vi "zad3.vi"() -> ()   [LabVIEW 2017]
panel:
  out "Numeric 2":dbl
  out "Numeric":dbl
  in  "Prąd [mA]":dbl min=0.0 max=1.1
  in  "TRYB":i16(knob) step=1 scale=1.0..3.0
  in  "DAC0":dbl(knob) scale=0.04..2.5
  out "Rs":dbl
  in  "Interval (ms)":u32=500
  in  "stop":bool
  out "AIN3":dbl format="%.6f"
  out "AIN2":dbl format="%.6f"
  out "Error Message":string
  out "error out":errorcluster
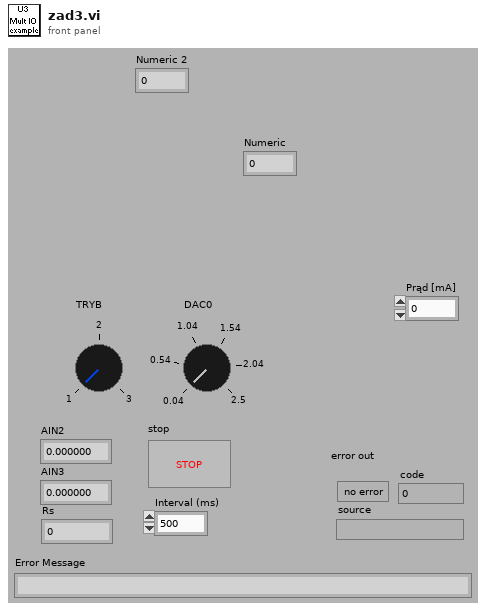
[diagram p1: front panel]
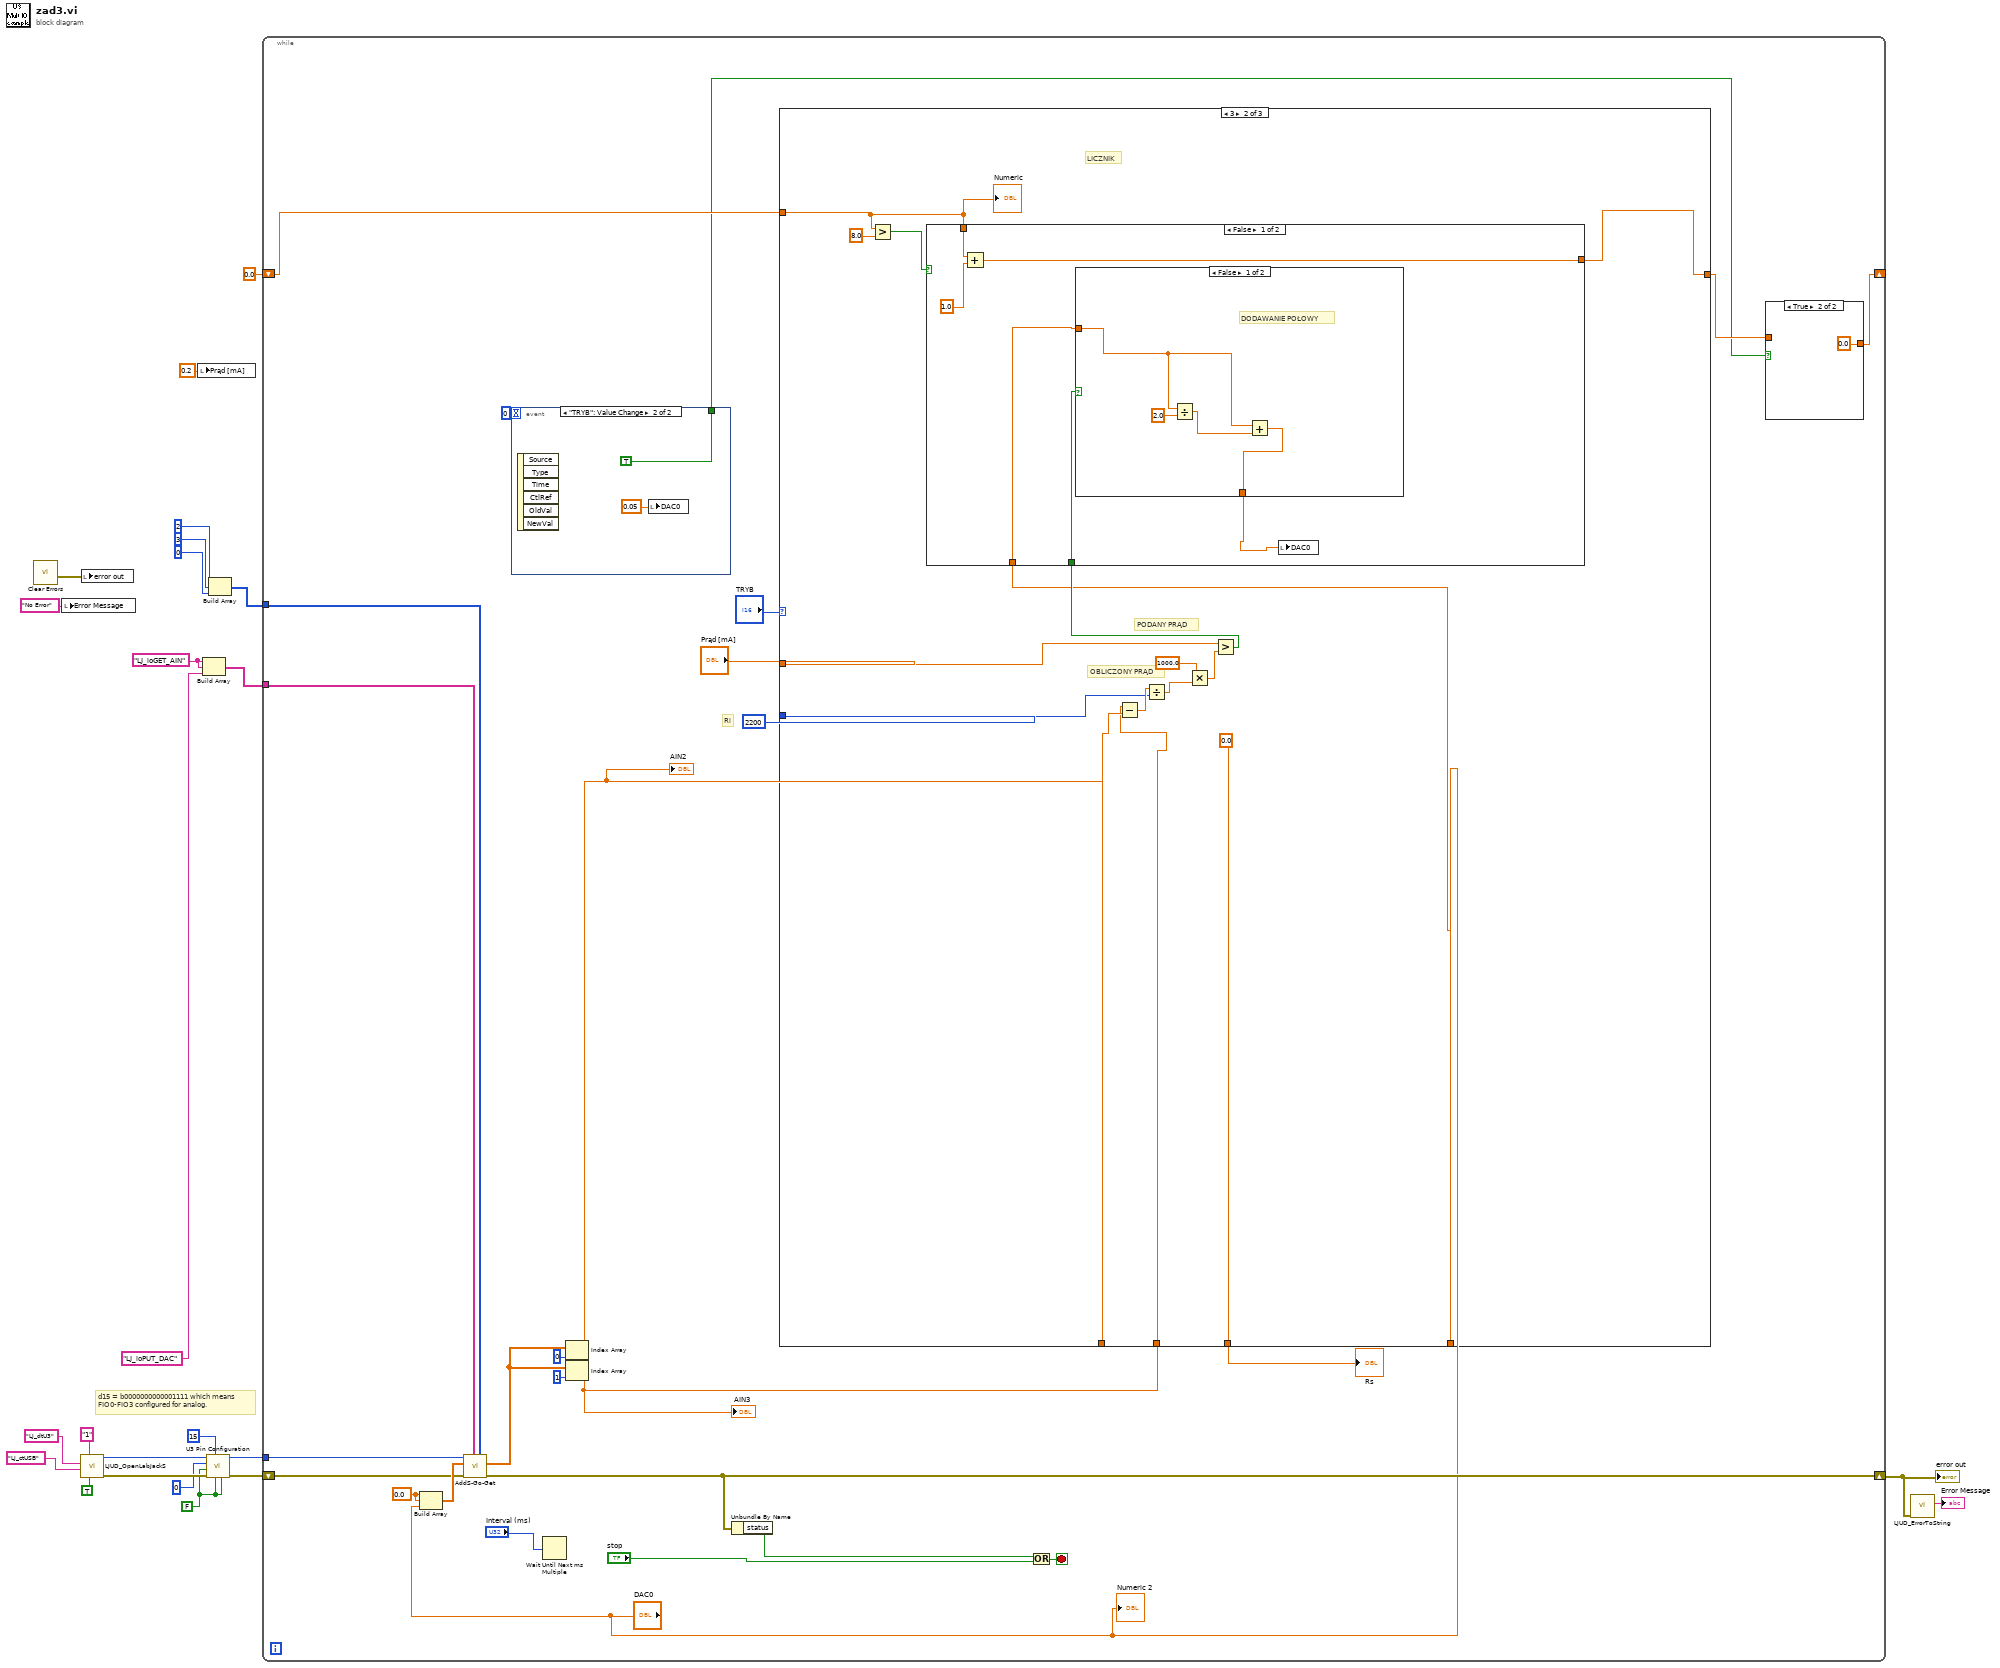
[diagram p0: block diagram]
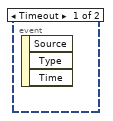
[diagram p3: hidden frame]
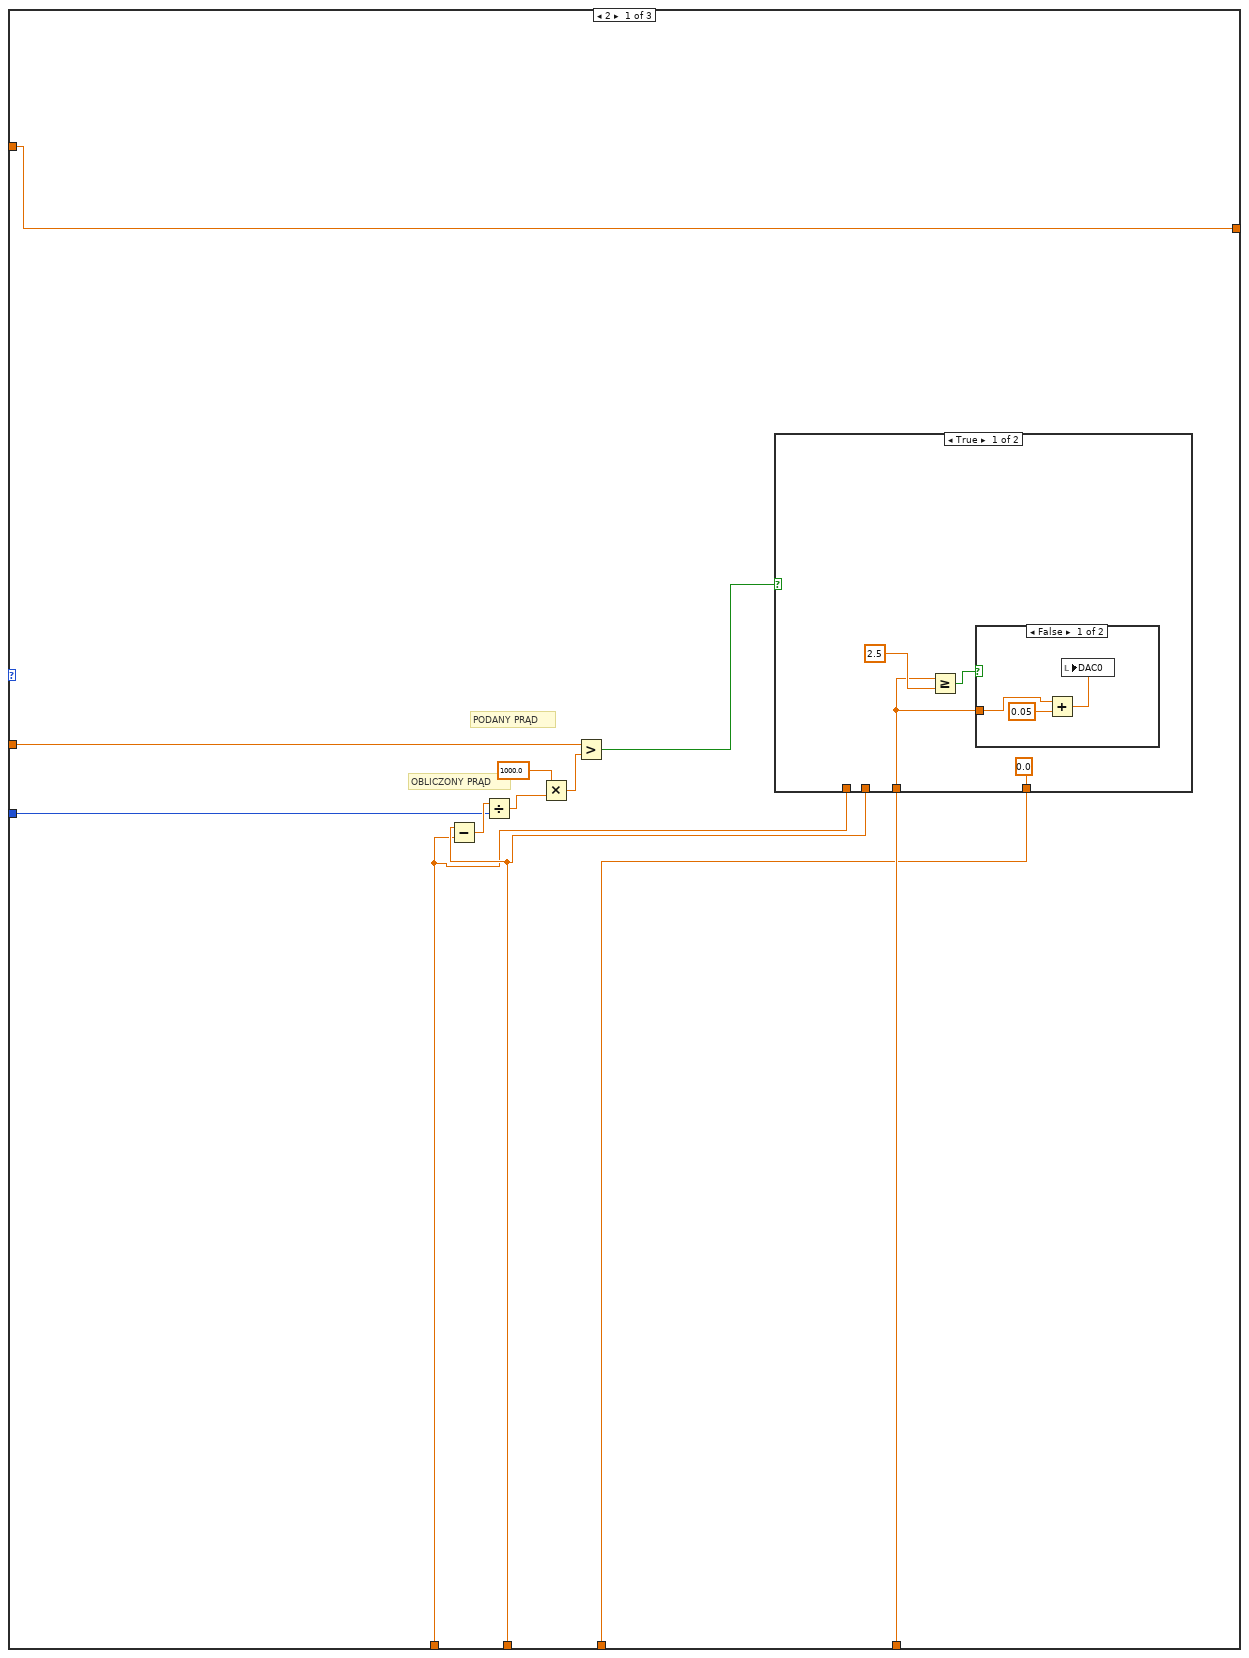
[diagram p4: hidden frame]
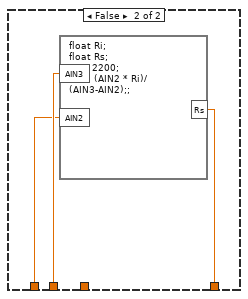
[diagram p6: hidden frame]
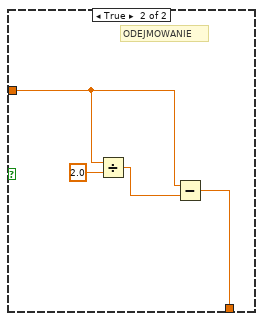
[diagram p7: hidden frame]
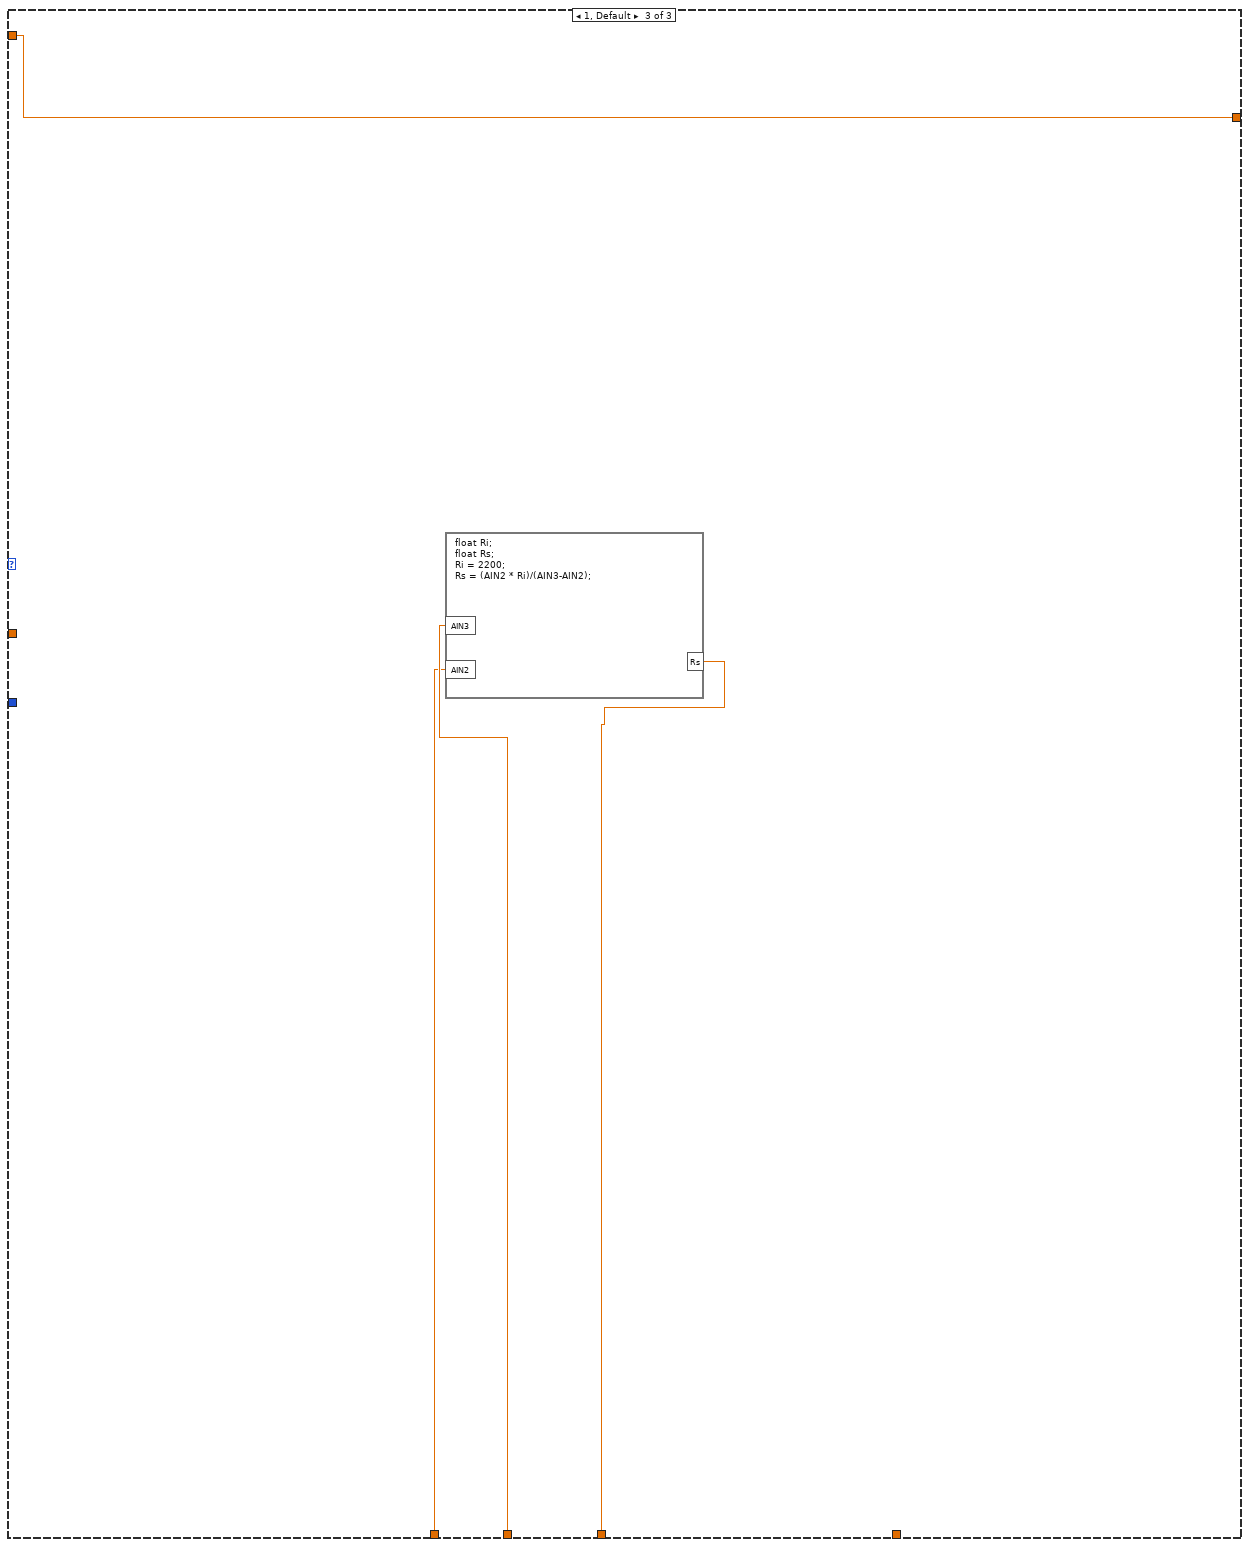
[diagram p9: hidden frame]
diagram:
  w7 = FALSE ("Enable DAC1")
  w3 = "LJ_ioGET_AIN" ("IOType")
  # "d15 = b0000000000001111 which means\nFIO0-FIO3 configured for analog."
  n1 = call <vilib>:"Clear Errors.vi"() -> ("error out"=w5:errorcluster)  [unwired: 6 in, 1 out]
  n2 = local write "Error Message"("No Error" ("Error Message")) -> ()
  n3 = call "LJUD_OpenLabJackS.vi"("FirstFound"=TRUE, "Address"="1", "ConnectionType"="LJ_ctUSB", "DeviceType"="LJ_dtU3") -> ("error out"=w12:errorcluster, "Handle"=w10:i32)  [unwired: 5 in, 1 out]
  n4 = local write "error out"(w5) -> ()
  n5 = local write "Prąd [mA]"(0.2 ("Prąd [A]")) -> ()
  n6 = Build Array(w3, w3, "LJ_ioPUT_DAC" ("IOType")) -> (w23:string[])
  n7 = call "U3 Pin Configuration.vi"("Enable Counter1"=w7, "Enable Counter0"=w7, "FIO/EIO Analog Enable"=15, "error in"=w12, "Enable DAC1"=w7, "Number of Timers Enabled"=u8 0, "Handle In"=w10) -> ("error out"=w13:errorcluster, "Handle Out"=w11:i32)  [unwired: 3 in]
  n8 = Build Array(2, 3, 0) -> (w22:i32[])
  n9 = while {
    shift-left: w13 -> [w39]
    shift-right: [w38] -> w14
    tunnel: w11 -> [w43]
    tunnel: w22 -> [w49]
    tunnel: w23 -> [w50]
    shift-right: [w27] -> _
    shift-left: 0.0 -> [w29]
    stop <- w42 stop-if-true
    w48 = 0.0 ("Input Element")
    # "Ri"
    n10 = Build Array(w48, w48, "DAC0") -> (w47:dbl[])
    n11 = call "AddS-Go-Get.vi"("Channels"=w49, "IOTypes"=w50, "error in"=w39, "Values Write"=w47, "Handle In"=w43) -> ("error out"=w38:errorcluster, "Values Read"=w44:dbl[])  [unwired: 4 in, 1 out]
    n12 = event shown="[1] \"TRYB\": Value Change" {
      selector: _ -> [_ _]
      dyn-events: _ -> [_ _]
      timeout: 0 -> [_ _]
      tunnel: [_ TRUE] -> w26
      event Timeout {
        n13 = event-data() -> ()  [unwired: 1 in, 3 out]
      }
      event "TRYB": Value Change {
        n14 = event-data() -> ()  [unwired: 1 in, 6 out]
        n15 = local write "DAC0"(0.05 ("DAC0")) -> ()
      }
    }
    n16 = Wait Until Next ms Multiple(millisecond multiple="Interval (ms)") -> ()  [unwired: 1 out]
    n17 = Index Array(array=w44, index=0 ("Index")) -> (element=w35:dbl)
    "AIN2" <- w35
    n18 = Index Array(array=w44, index=1 ("Index")) -> (element=w36:dbl)
    "AIN3" <- w36
    n19 = Unbundle By Name(w38) -> ("status"=w40:bool)
    n20 = case shown="3" "TRYB" {
      tunnel: w36 -> [w62 w85 w110]
      tunnel: w35 -> [w61 w86 w109]
      tunnel: [w60 0.0 w108] -> w34
      tunnel: 2200 -> [w65 w87 _]
      tunnel: "DAC0" -> [w63 w78 _]
      tunnel: "Prąd [mA]" -> [w56 w83 _]
      tunnel: [w55 w80 w107] -> w28
      tunnel: w29 -> [w55 w81 w107]
      frame 2 {
        # "PODANY PRĄD"
        # "OBLICZONY PRĄD"
        n21 = Subtract(x=w62, y=w61) -> (x-y=w66:dbl)
        n22 = Divide(x=w66, y=w65) -> (x/y=w59:dbl)
        n23 = Multiply(x=1000.0, y=w59) -> (x*y=w57:dbl)
        n24 = Greater?(x=w56, y=w57) -> (0:w64:bool)
        n25 = case shown="True" w64 {
          tunnel: w63 -> [w68 _]
          tunnel: w62 -> [_ w76]
          tunnel: w61 -> [_ w75]
          tunnel: [0.0 w74] -> w60
          frame True {
            n26 = Greater Or Equal?(x=w68, y=2.5) -> (x >= y?=w69:bool)
            n27 = case shown="False" w69 {
              tunnel: w68 -> [w71 _]
              frame False {
                n28 = Add(x=w71, y=0.05) -> (x+y=w73:dbl)
                n29 = local write "DAC0"(w73) -> ()
              }
              frame True {
              }
            }
          }
          frame False {
            n30 = formula code="float Ri;\nfloat Rs;\nRi = 2200;\nRs = (AIN2 * Ri)/(AIN3-AIN2);;"("AIN3"=w76, "AIN2"=w75) -> ("Rs"=w74:dbl)
          }
        }
      }
      frame 3 {
        # "LICZNIK"
        # "PODANY PRĄD"
        # "OBLICZONY PRĄD"
        n31 = Greater?(x=w81, y=8.0) -> (0:w77:bool)
        n32 = Subtract(x=w85, y=w86) -> (x-y=w91:dbl)
        n33 = Divide(x=w91, y=w87) -> (x/y=w90:dbl)
        n34 = Multiply(x=1000.0, y=w90) -> (x*y=w88:dbl)
        n35 = Greater?(x=w83, y=w88) -> (0:w79:bool)
        n36 = case shown="False" w77 {
          tunnel: w81 -> [w96 w106]
          tunnel: [w95 w106] -> w80
          tunnel: w79 -> [w94 _]
          tunnel: w78 -> [w93 _]
          frame False {
            n37 = Add(x=w96, y=1.0) -> (x+y=w95:dbl)
            n38 = case shown="False" w94 {
              tunnel: w93 -> [w100 w104]
              tunnel: [w98 w102] -> w92
              frame False {
                # "DODAWANIE POŁOWY"
                n39 = Divide(x=w100, y=2.0) -> (x/y=w99:dbl)
                n40 = Add(x=w100, y=w99) -> (x+y=w98:dbl)
              }
              frame True {
                # "ODEJMOWANIE"
                n41 = Divide(x=w104, y=2.0) -> (x/y=w103:dbl)
                n42 = Subtract(x=w104, y=w103) -> (x-y=w102:dbl)
              }
            }
            n43 = local write "DAC0"(w92) -> ()
          }
          frame True {
          }
        }
        "Numeric" <- w81
      }
      frame 1, Default {
        n44 = formula code="float Ri;\nfloat Rs;\nRi = 2200;\nRs = (AIN2 * Ri)/(AIN3-AIN2);"("AIN3"=w110, "AIN2"=w109) -> ("Rs"=w108:dbl)
      }
    }
    "Rs" <- w34
    n45 = Or(x=w40, y="stop") -> (x .or. y?=w42:bool)
    n46 = case shown="True" w26 {
      tunnel: w28 -> [w51 _]
      tunnel: [w51 0.0] -> w27
      frame False {
      }
      frame True {
      }
    }
    "Numeric 2" <- "DAC0"
  }
  "error out" <- w14
  n47 = call "LJUD_ErrorToString.vi"("error in"=w14) -> ("String"=→"Error Message":string)  [unwired: 10 in]
